vi "R30_1-FPGA.vi"() -> ()   [LabVIEW 2016]
uses:
  Glassman Control.ctl
  Faraday Cup Readback.ctl
  Aperture Readback.ctl
  Gate Valve Readback.ctl
  Glassman Readback.ctl
  <vilib>/LabVIEW Targets/FPGA/cRIO/shared/nicrio_ModuleControls/nicrio_cRIO-9871_BaudRateEnum.ctl
  <vilib>/LabVIEW Targets/FPGA/cRIO/shared/nicrio_ModuleControls/nicrio_cRIO-9871_ParityEnum.ctl
  <vilib>/LabVIEW Targets/FPGA/cRIO/shared/nicrio_ModuleControls/nicrio_cRIO-9871_StopBitsEnum.ctl
  <vilib>/LabVIEW Targets/FPGA/cRIO/shared/nicrio_ModuleControls/nicrio_cRIO-9871_DataBitsEnum.ctl
  <vilib>/Platform/TimedLoop/XDataNode/timing_clust.ctl
  <vilib>/Platform/TimedLoop/XDataNode/nitl_modes.ctl
  <vilib>/Platform/TimedLoop/XDataNode/wakeup.ctl
  <vilib>/rvi/FXPMathLib/basic elements/FxpIntAccumulator/subVIs/nifxpmath_IntAccumulator_SimConfig.ctl
  <vilib>/rvi/Emulation/niFpgaGetClockAttributes.vi
  <vilib>/rvi/Emulation/niFpgaSctlEmulationGetInTimedLoop.vi
  <vilib>/rvi/Emulation/niFpgaEmulationReportErrorSimple.vi
  <vilib>/rvi/eio/common/nirviEmuTemplateMethod_errors.vi
  <vilib>/rvi/Analysis/common/codeGenErrors/XNode/niFpgaXNodeCodeGenErrorHandle.vi
  <vilib>/rvi/Emulation/niFpgaCriticalErrorInLSC.vi
  <vilib>/rvi/FXPMathLib/basic elements/FxpIntAccumulator/simVIs/DllFxpIntAccumulator_sub.vi
  <vilib>/rvi/eio/common/nirviEmuTemplatePropertySet_errors.vi
  <vilib>/eio/EIONode/EIONode.xnode
  <vilib>/rvi/Analysis/measure/dc-rms/XNode/niFpgaDC-RMS.xnode
  <vilib>/Platform/TimedLoop/XDataNode/XDataNode.xnode
  <vilib>/rvi/FXPMathLib/basic elements/FxpIntAccumulator/XNode/nifxpmath_IntAccumulator.xnode
  <vilib>/rvi/FXPMathLib/FxpMul/XNode/nifxpmath_Multiplier.xnode
  <vilib>/eio/EIOPropertyNode/EIOPropertyNode.xnode
  <vilib>/eio/EIOMethodNode/EIOMethodNode.xnode
  <vilib>/Platform/TimedLoop/XDataNode/XDNodeRunTimeDep.lvlib
  <vilib>/rvi/FXPMathLib/sim/FxpSim.dll
  <vilib>/rvi/eio/common/nirviEmuTemplatePropertyGet_errors.vi
  <vilib>/rvi/eio/common/nirviEmuTemplatePropertyGet_noerrors.vi
  <vilib>/rvi/eio/common/nirviEmuTemplatePropertySet_noerrors.vi
panel:
  in  "Switch Obj Vac interlock bypass":bool
  in  "Vac cluster 3 interlock bypass":bool
  in  "Vac cluster 2 interlock bypass":bool
  in  "Vac cluster 1 interlock bypass":bool
  in  "Switch Object Vac Interlock":bool
  out "HV readback loop error":errorcluster
  out "Quad B I read":fxp<+/-,26,5>
  out "Quad A I read":fxp<+/-,26,5>
  out "ESA- Monitor":T1
  out "Mag Steerer Monitor":T1
  out "Y- Steerer Monitor":T1
  out "ESA+ Monitor":T1
  out "X+ Steerer Monitor":T1
  out "X- Steerer Monitor":T1
  out "Y+ Steerer Monitor":T1
  in  "RT error":bool
  out "GV Interlock loop error":errorcluster
  out "Vac cluster 3 Interlock":bool
  out "Vac cluster 2 Interlock":bool
  out "Vac cluster 1 Interlock":bool
  in  "Turbo 2 GV Actuator":bool
  in  "Beamline GV 2 Actuator":bool
  in  "Cryo Pump GV Actuator":bool
  in  "Beamline GV 1 Actuator":bool
  in  "Turbo 1 GV Actuator":bool
  in  "Switch Magnet GV Actuator":bool
  out "GV Status Loop error":errorcluster
  out "Cryo Pump GV Status":T2
  out "Turbo 2 GV Status":T2
  out "Beamline GV 2 Status":T2
  out "Turbo 1 GV Status":T2
  out "Beamline GV 1 Status":T2
  out "Switching Mag GV Status":T2
  in  "ESA- HV Enable":bool
  in  "ESA+ HV Enable":bool
  out "Switch Magnet Aperture Position":T3
  out "Detector Aperture Position":T3
  out "Detector FC Position":T4
  out "Switch Magnet FC Position":T4
  out "Actuator loop error":errorcluster
  in  "Y- Steerer V set":T5
  in  "Y+ Steerer V set":T5
  in  "X- Steerer V set":T5
  in  "X+ Steerer V set":T5
  in  "Quad B set":fxp<+/-,20,5>
  in  "Quad A set":fxp<+/-,20,5>
  in  "ESA Voltage set":fxp<+/-,20,5>
  out "HV control loop error":errorcluster
  out "Cryo Readback error":errorcluster
  out "Vacuum Gauge 1 error":errorcluster
  out "Vacuum Gauge 2 error":errorcluster
  out "Vacuum Gauge 3 error":errorcluster
  out "Switch Image Ion Gauge 1":u8[](array[numeric])
  out "Switch Image Convectron 1":u8[](array[numeric])
  out "Time since repurge":u8[](array[numeric])
  out "1st stage temp":u8[](array[numeric])
  out "2nd stage temp":u8[](array[numeric])
  out "Cryo On-time":u8[](array[numeric])
  out "Cryo Status":u8[](array[numeric])
  out "R30 ESA Convectron  1":u8[](array[numeric])
  out "R30 ESA Ion gauge 1":u8[](array[numeric])
  out "R30 Detector Convectron  1":u8[](array[numeric])
  out "R30 Detector Ion gauge 1":u8[](array[numeric])
  in  "Mag Steerer I-program":fxp<+/-,20,5> format="%.17g"
  in  "Switch magnet Aperture Actuator":bool
  in  "Detector Aperture Actuator":bool
  in  "Detector FC Actuator":bool
  in  "Switch magnet FC Actuator":bool
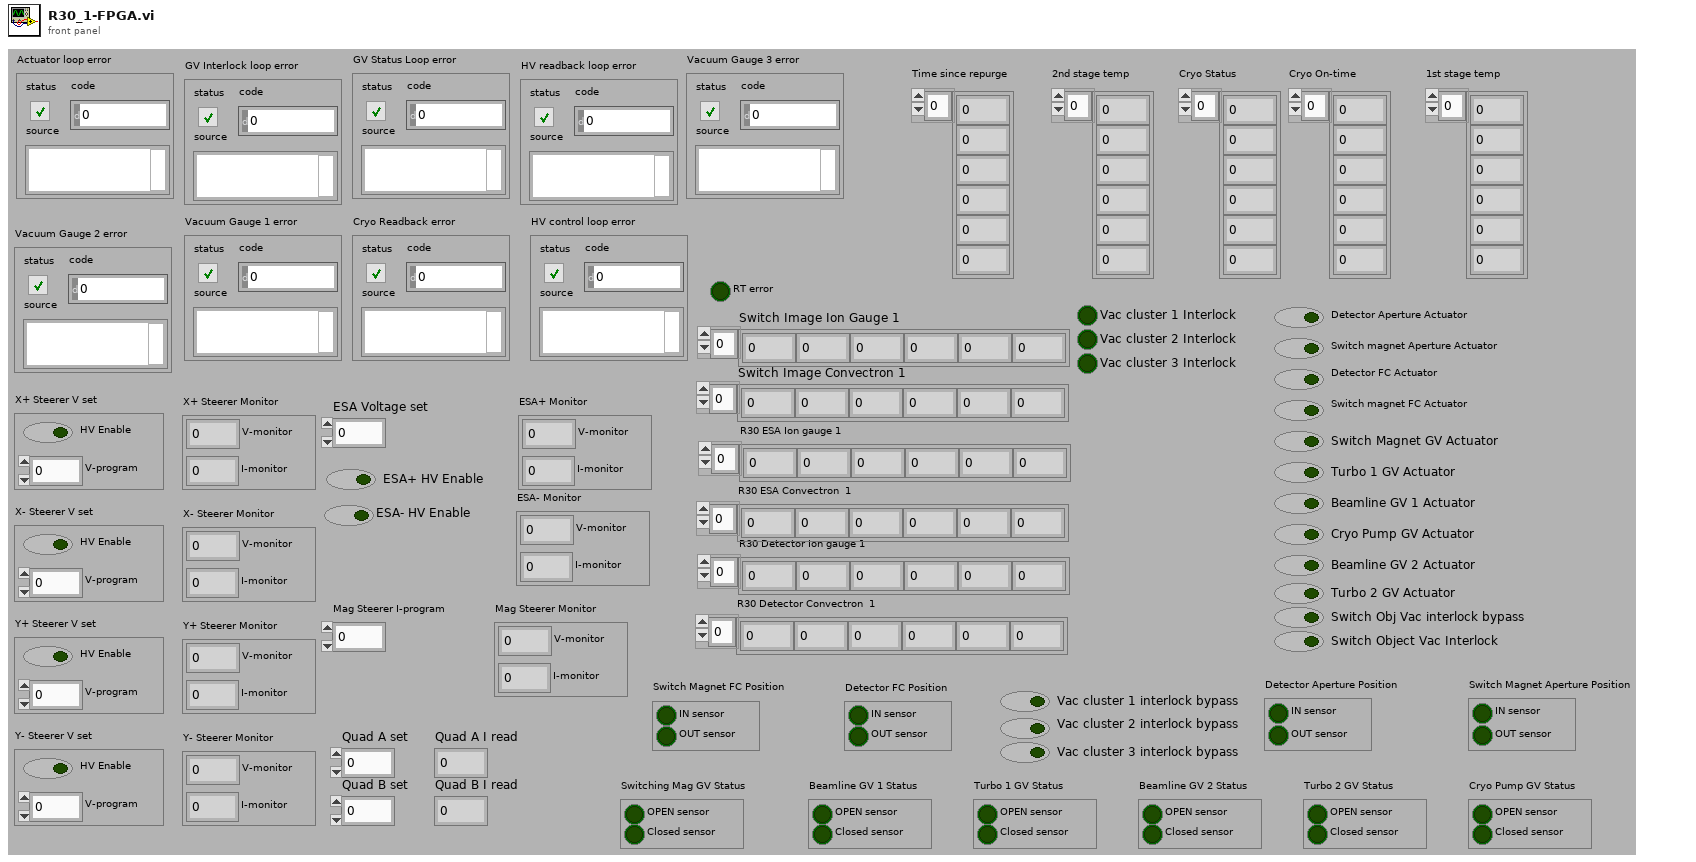
[diagram p1: front panel]
types:
  T1 = typedef "Glassman Readback.ctl" = cluster{"I-monitor":fxp<+/-,16,5>, "V-monitor":fxp<+/-,16,5>}
  T2 = typedef "Gate Valve Readback.ctl" = cluster{"OPEN sensor":bool, "Closed sensor":bool}
  T3 = typedef "Aperture Readback.ctl" = cluster{"IN sensor":bool, "OUT sensor":bool}
  T4 = typedef "Faraday Cup Readback.ctl" = cluster{"IN sensor":bool, "OUT sensor":bool}
  T5 = typedef "Glassman Control.ctl" = cluster{"V-program":fxp<+/-,16,5>, "HV Enable":bool}
  T6 = typedef "nicrio_cRIO-9871_StopBitsEnum.ctl" = enum8{"1", "1.5", "2"}
  T7 = typedef "nicrio_cRIO-9871_ParityEnum.ctl" = enum8{"None", "Odd", "Even", "Mark", "Space"}
  T8 = typedef "nicrio_cRIO-9871_DataBitsEnum.ctl" = enum8{"5", "6", "7", "8"}
  T9 = typedef "nicrio_cRIO-9871_BaudRateEnum.ctl" = enum16{"75 bps", "110 bps", "134 bps", "150 bps", "300 bps", "600 bps", "1200 bps", "1800 bps", "2400 bps", "4800 bps", "7200 bps", "9600 bps", "14.4 kbps", "19.2 kbps", "28.8 kbps", "38.4 kbps", "57.6 kbps", "115.2 kbps", "230.4 kbps", "460.8 kbps", "921.6 kbps"}
  T10 = typedef "XDNodeRunTimeDep.lvlib/timing_clust.ctl" = cluster{"Expected End [f-1]":u64, "Actual End [f-1]":u64, "Finished Late? [f-1]":bool, "Expected End [i-1]":u64, "Actual End [i-1]":u64, "Finished Late? [i-1]":bool, "Expected Start [i]":u64, "Actual Start [i]":u64, "Expected Start [f]":u64, "Actual Start [f]":u64, "Source Name":string, "Structure Name":string, "Period":i64, "Deadline":i64, "Offset":i64, "Start":i64, "Priority":i32, "Timeout":i32, "Mode":T11, "Wakeup Reason":T12, "Error":errorcluster, "Source Type":string, "Secondary Source Type":string, "Global End Time":u64, "Global Start Time":u64, "Frame Duration":u64, "Iteration Duration":u64, "Assigned CPU":i32, "I/O Scan Engine Mode":u32}
  T11 = typedef "XDNodeRunTimeDep.lvlib/nitl_modes.ctl" = enum32{"No Change", "Process missed periods, maintain original phase", "Discard missed periods, maintain original phase", "Process missed periods, ignore original phase", "Discard missed periods, ignore original phase"}
  T12 = typedef "XDNodeRunTimeDep.lvlib/wakeup.ctl" = enum32{"Normal", "Aborted", "Asynchronous wakeup", "Timing source error", "Timed loop error", "Timeout"}
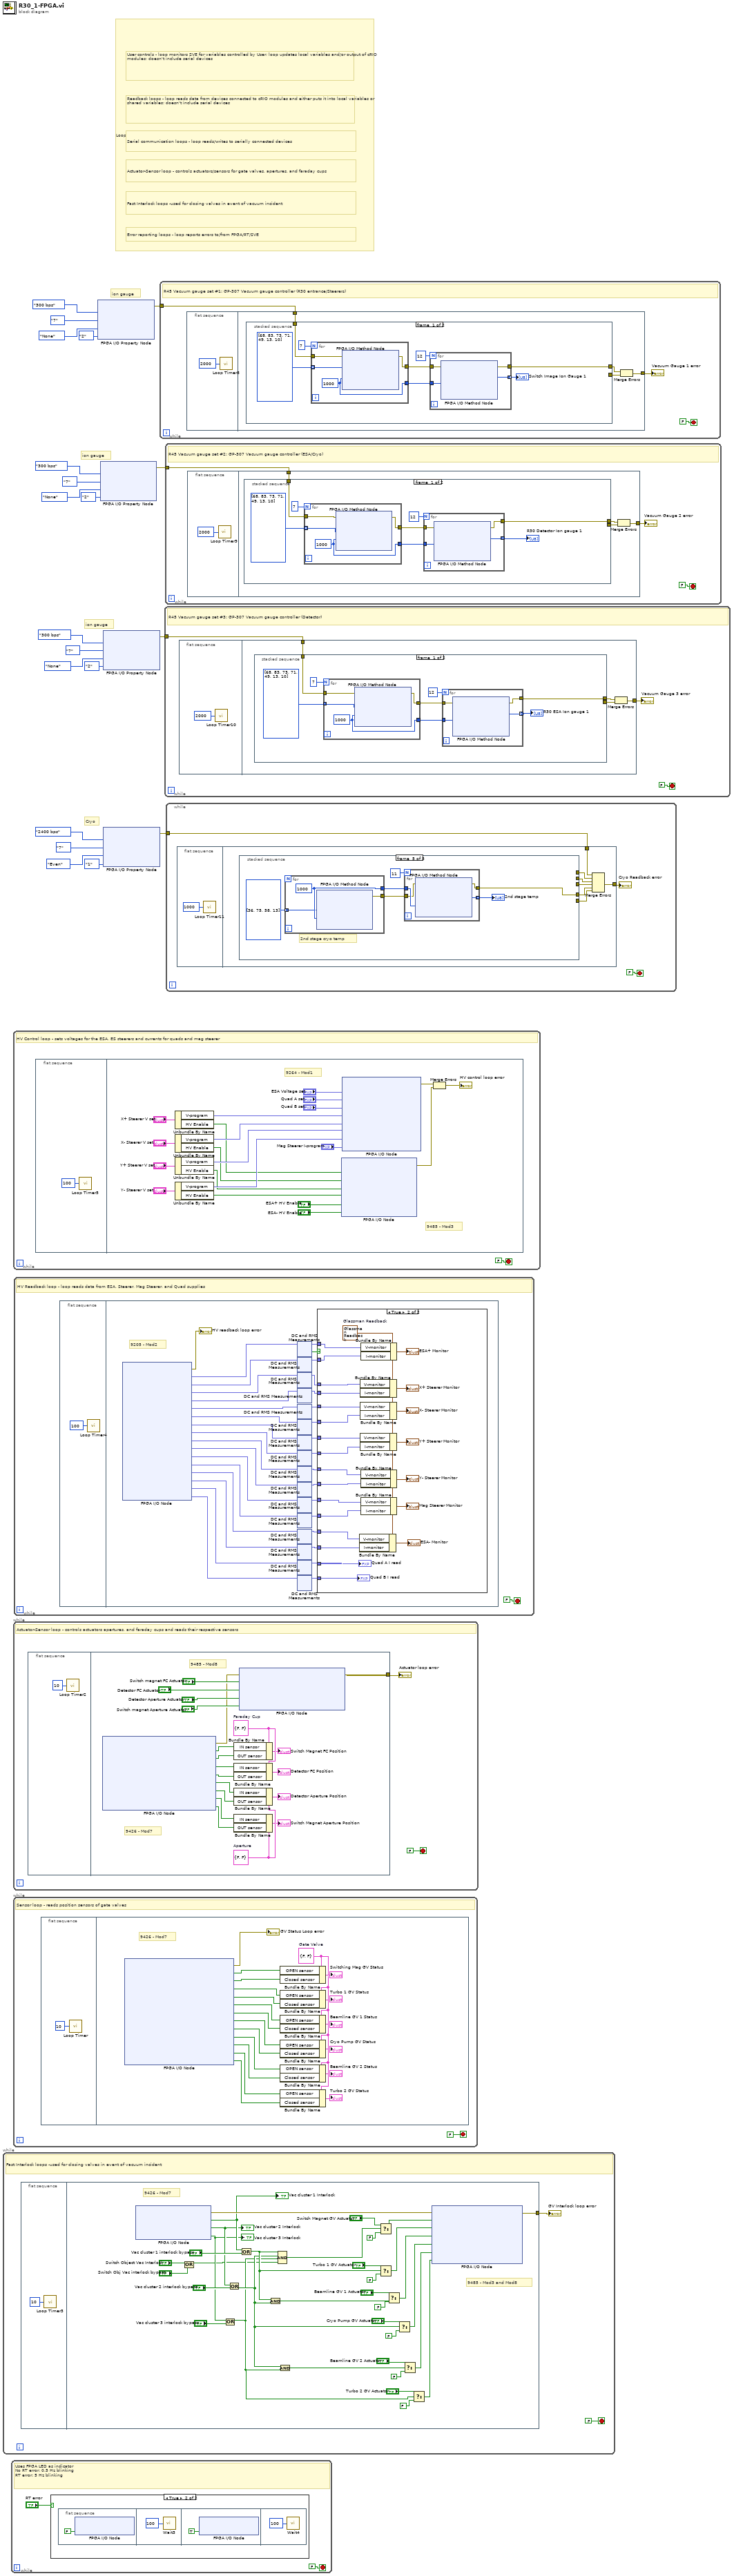
[diagram p0: block diagram]
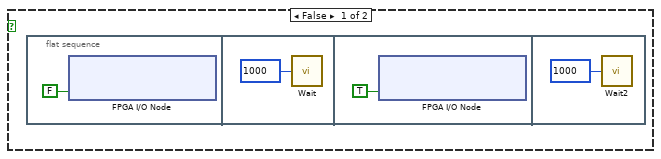
[diagram p2: hidden frame]
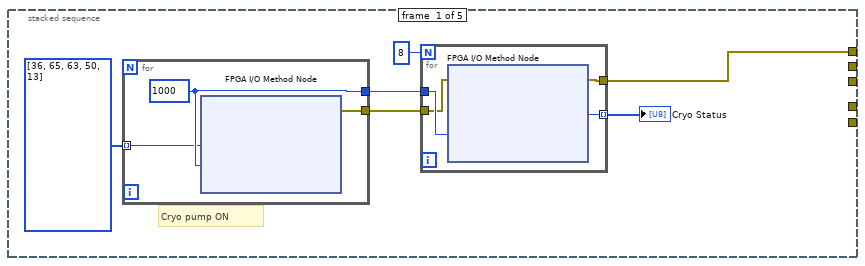
[diagram p3: hidden frame]
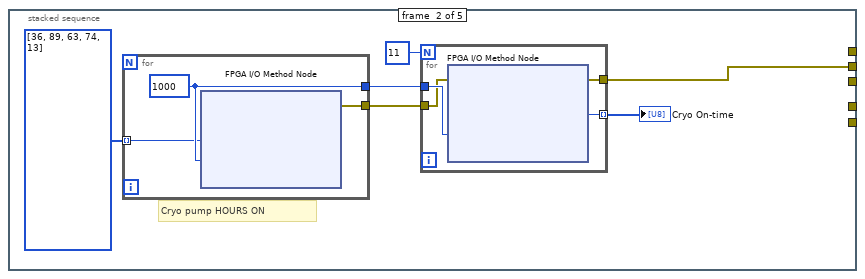
[diagram p4: hidden frame]
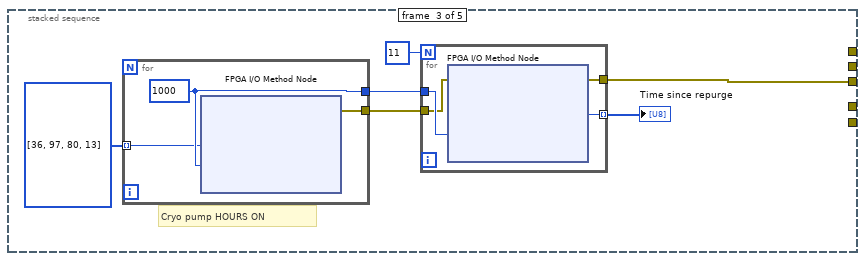
[diagram p5: hidden frame]
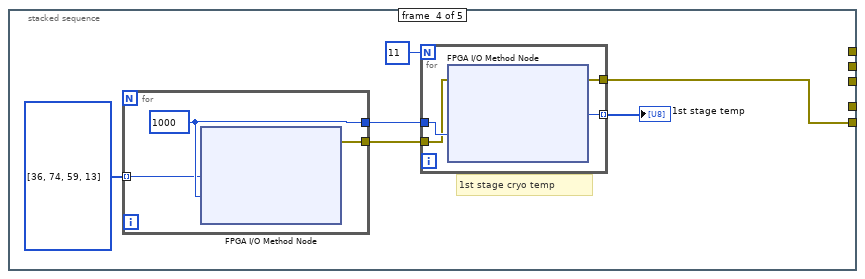
[diagram p6: hidden frame]
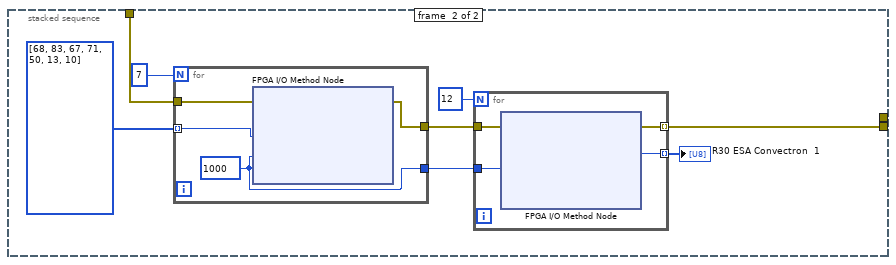
[diagram p7: hidden frame]
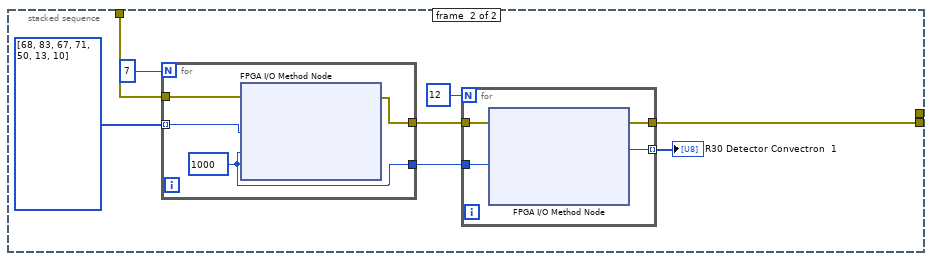
[diagram p8: hidden frame]
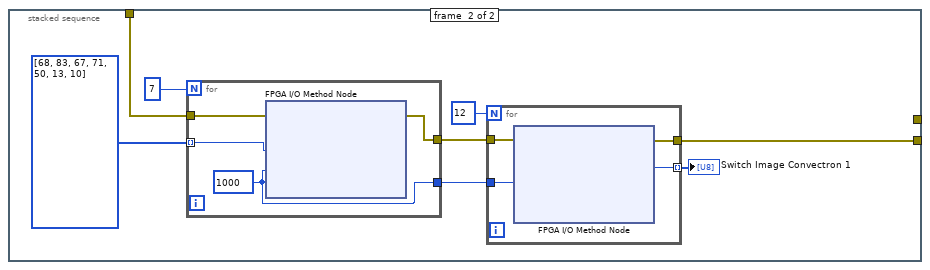
[diagram p9: hidden frame]
diagram:
  # "Actuator-Sensor loop - controls actuators/sensors for gate valves, apertures, and faraday cups"
  # "Fast Interlock loops -used for closing valves in event of vacuum incident"
  # "Error reporting loops - loop reports errors to/from FPGA/RT/SVE"
  # "Serial communication loops - loop reads/writes to serially connected devices"
  # "Readback loops - loop reads data from devices connected to cRIO modules and either puts it into local variables or shared variables; doesn't include serial devices"
  # "User controls - loop monitors SVE for variables controlled by User; loop updates local variables and/or output of cRIO modules; doesn't include serial devices"
  # "Loop legend - loops are color coded by responsibility"
  # "Cryo"
  # "ion gauge"
  # "ion gauge"
  # "ion gauge"
  n1 = while {
    stop <- FALSE stop-if-true
    # "Fast Interlock loops -used for closing valves in event of vacuum incident"
    n2 = flat-sequence {
      tunnel: [w36] -> w21
      frame #0 {
        n3 = call "Loop Timer3"("Count(uSec)"=u32 10) -> ()  [unwired: 1 out]
      }
      frame #1 {
        # "9485 - Mod3 and Mod8"
        # "9426 - Mod7"
        n4 = xnode "FPGA I/O Node"() -> ("error out"=w58:errorcluster, "Vac cluster 1 Interlock"=w33:bool, "Vac cluster 2 Interlock"=w30:bool, "Vac cluster 3 Interlock"=w28:bool)  [unwired: 4 in, 3 out]
        "Vac cluster 1 Interlock" <- w33
        "Vac cluster 2 Interlock" <- w30
        "Vac cluster 3 Interlock" <- w28
        n5 = Or(x="Switch Object Vac Interlock", y="Switch Obj Vac interlock bypass") -> (x .or. y?=w25:bool)
        n6 = Or(x=w28, y="Vac cluster 3 interlock bypass") -> (x .or. y?=w27:bool)
        n7 = Or(x=w30, y="Vac cluster 2 interlock bypass") -> (x .or. y?=w31:bool)
        n8 = Or(x=w33, y="Vac cluster 1 interlock bypass") -> (x .or. y?=w34:bool)
        n9 = And(x=w34, y=w31) -> (x .and. y?=w44:bool)
        n10 = Compound Arithmetic op=AND(w34, w31, w27, w25) -> (w38:bool)
        n11 = And(x=w31, y=w27) -> (x .and. y?=w51:bool)
        n12 = Select(t="Switch Magnet GV Actuator", s=w38, f=FALSE) -> (s? t:f=w37:bool)
        n13 = Select(t="Turbo 1 GV Actuator", s=w34, f=FALSE) -> (s? t:f=w42:bool)
        n14 = Select(t="Beamline GV 1 Actuator", s=w44, f=FALSE) -> (s? t:f=w46:bool)
        n15 = Select(t="Cryo Pump GV Actuator", s=w31, f=FALSE) -> (s? t:f=w49:bool)
        n16 = Select(t="Beamline GV 2 Actuator", s=w51, f=FALSE) -> (s? t:f=w53:bool)
        n17 = Select(t="Turbo 2 GV Actuator", s=w27, f=FALSE) -> (s? t:f=w56:bool)
        n18 = xnode "FPGA I/O Node"("error in"=w58, "Switch Magnet GV Actuator"=w37, "Turbo 1 GV Actuator"=w42, "Beamline GV 1 Actuator"=w46, "Cryo Pump GV Actuator"=w49, "Beamline GV 2 Actuator"=w53, "Turbo 2 GV Actuator"=w56) -> ("error out"=w36:errorcluster)  [unwired: 6 in, 6 out]
      }
    }
    "GV Interlock loop error" <- w21
  }
  n19 = while {
    stop <- FALSE stop-if-true
    # "Uses FPGA LED as indicator\nNo RT error: 0.5 Hz blinking\nRT error: 5 Hz blinking"
    n20 = case shown="True" "RT error" {
      frame False {
        n21 = flat-sequence {
          frame #0 {
            n22 = xnode "FPGA I/O Node"("USER FPGA LED"=FALSE ("FPGA LED")) -> ()  [unwired: 1 in, 1 out]
          }
          frame #1 {
            n23 = call "Wait"("Count(mSec)"=u16 1000) -> ()  [unwired: 1 out]
          }
          frame #2 {
            n24 = xnode "FPGA I/O Node"("USER FPGA LED"=TRUE ("FPGA LED")) -> ()  [unwired: 1 in, 1 out]
          }
          frame #3 {
            n25 = call "Wait2"("Count(mSec)"=u16 1000) -> ()  [unwired: 1 out]
          }
        }
      }
      frame True {
        n26 = flat-sequence {
          frame #0 {
            n27 = xnode "FPGA I/O Node"("USER FPGA LED"=FALSE ("FPGA LED")) -> ()  [unwired: 1 in, 1 out]
          }
          frame #1 {
            n28 = call "Wait3"("Count(mSec)"=u16 100) -> ()  [unwired: 1 out]
          }
          frame #2 {
            n29 = xnode "FPGA I/O Node"("USER FPGA LED"=TRUE ("FPGA LED")) -> ()  [unwired: 1 in, 1 out]
          }
          frame #3 {
            n30 = call "Wait4"("Count(mSec)"=u16 100) -> ()  [unwired: 1 out]
          }
        }
      }
    }
  }
  n31 = while {
    stop <- FALSE stop-if-true
    # "Actuator-Sensor loop - controls actuators apertures, and faraday cups and reads their respective sensors"
    n32 = flat-sequence {
      tunnel: [w89] -> w69
      frame #0 {
        n33 = call "Loop Timer2"("Count(uSec)"=u32 10) -> ()  [unwired: 1 out]
      }
      frame #1 {
        w78 = T3 {"IN sensor"=FALSE, "OUT sensor"=FALSE}  # Aperture
        w81 = T4 {"IN sensor"=FALSE, "OUT sensor"=FALSE}  # Faraday Cup
        # "9485 - Mod8"
        # "9426 - Mod7"
        n34 = xnode "FPGA I/O Node"() -> ("error out"=w86:errorcluster, "Switch Magnet FC IN sensor"=w85:bool, "Switch Magnet FC OUT sensor"=w84:bool, "Detector FC IN sensor"=w83:bool, "Detector FC OUT sensor"=w82:bool, "Detector Aperture IN sensor"=w74:bool, "Detector Aperture OUT sensor"=w75:bool, "Switch Magnet Aperture IN sensor"=w76:bool, "Switch Magnet Aperture OUT sensor"=w77:bool)  [unwired: 9 in, 8 out]
        n35 = Bundle By Name(cluster=w81, "IN sensor"=w85, "OUT sensor"=w84) -> (→"Switch Magnet FC Position":T4)
        n36 = Bundle By Name(cluster=w81, "IN sensor"=w83, "OUT sensor"=w82) -> (→"Detector FC Position":T4)
        n37 = Bundle By Name(cluster=w78, "IN sensor"=w74, "OUT sensor"=w75) -> (→"Detector Aperture Position":T3)
        n38 = Bundle By Name(cluster=w78, "IN sensor"=w76, "OUT sensor"=w77) -> (→"Switch Magnet Aperture Position":T3)
        n39 = xnode "FPGA I/O Node"("error in"=w86, "Switch Magnet FC Actuator"="Switch magnet FC Actuator", "Detector FC Actuator"="Detector FC Actuator", "Detector Aperture Actuator"="Detector Aperture Actuator", "Switch Magnet Aperture Actuator"="Switch magnet Aperture Actuator") -> ("error out"=w89:errorcluster)  [unwired: 4 in, 4 out]
      }
    }
    "Actuator loop error" <- w69
  }
  n40 = while {
    stop <- FALSE stop-if-true
    # "Sensor loop - reads position sensors of gate valves"
    n41 = flat-sequence {
      frame #0 {
        n42 = call "Loop Timer"("Count(uSec)"=u32 10) -> ()  [unwired: 1 out]
      }
      frame #1 {
        w112 = T2 {"OPEN sensor"=FALSE, "Closed sensor"=FALSE}  # Gate Valve
        # "9426 - Mod7"
        n43 = xnode "FPGA I/O Node"() -> ("error out"=→"GV Status Loop error":errorcluster, "Swtich Magnet GV OPEN Sensor"=w111:bool, "Swtich Magnet GV CLOSED Sensor"=w110:bool, "Turbo 1 GV OPEN sensor"=w109:bool, "Turbo 1 GV CLOSED sensor"=w108:bool, "Beamline GV 1 OPEN sensor"=w107:bool, "Beamline GV 1 CLOSED sensor"=w106:bool, "Cryo Pump GV OPEN sensor"=w105:bool, "Cryo Pump GV CLOSED sensor"=w104:bool, "Beamline GV 2 OPEN sensor"=w103:bool, "Beamline GV 2 CLOSED sensor"=w102:bool, "Turbo 2 GV OPEN sensor"=w101:bool, "Turbo 2 GV CLOSED sensor"=w100:bool)  [unwired: 13 in, 12 out]
        n44 = Bundle By Name(cluster=w112, "OPEN sensor"=w111, "Closed sensor"=w110) -> (→"Switching Mag GV Status":T2)
        n45 = Bundle By Name(cluster=w112, "OPEN sensor"=w109, "Closed sensor"=w108) -> (→"Turbo 1 GV Status":T2)
        n46 = Bundle By Name(cluster=w112, "OPEN sensor"=w107, "Closed sensor"=w106) -> (→"Beamline GV 1 Status":T2)
        n47 = Bundle By Name(cluster=w112, "OPEN sensor"=w105, "Closed sensor"=w104) -> (→"Cryo Pump GV Status":T2)
        n48 = Bundle By Name(cluster=w112, "OPEN sensor"=w103, "Closed sensor"=w102) -> (→"Beamline GV 2 Status":T2)
        n49 = Bundle By Name(cluster=w112, "OPEN sensor"=w101, "Closed sensor"=w100) -> (→"Turbo 2 GV Status":T2)
      }
    }
  }
  n50 = while {
    stop <- FALSE stop-if-true
    # "HV Control loop - sets voltages for the ESA, ES steerers and currents for quads and mag steerer"
    n51 = flat-sequence {
      frame #0 {
        n52 = call "Loop Timer5"("Count(mSec)"=u32 100) -> ()  [unwired: 1 out]
      }
      frame #1 {
        # "9264 - Mod1"
        # "9485 - Mod3"
        n53 = Unbundle By Name("X+ Steerer V set") -> ("V-program"=w127:fxp<+/-,16,5>, "HV Enable"=w120:bool)
        n54 = Unbundle By Name("X- Steerer V set") -> ("V-program"=w126:fxp<+/-,16,5>, "HV Enable"=w121:bool)
        n55 = Unbundle By Name("Y+ Steerer V set") -> ("V-program"=w125:fxp<+/-,16,5>, "HV Enable"=w122:bool)
        n56 = Unbundle By Name("Y- Steerer V set") -> ("V-program"=w124:fxp<+/-,16,5>, "HV Enable"=w123:bool)
        n57 = xnode "FPGA I/O Node"("X+ Steerer HV Enable"=w120, "X- Steerer HV Enable"=w121, "Y+ Steerer HV Enable"=w122, "Y- Steerer HV Enable"=w123, "ESA+ HV Enable"="ESA+ HV Enable", "ESA- HV Enable"="ESA- HV Enable") -> ("error out"=w118:errorcluster)  [unwired: 7 in, 6 out]
        n58 = xnode "FPGA I/O Node"("ESA Voltage set"="ESA Voltage set", "Quad A set"="Quad A set", "Quad B set"="Quad B set", "X+ Steerer V set"=w127, "X- Steerer V set"=w126, "Y+ Steerer V set"=w125, "Y- Steerer V set"=w124, "Mag Steerer I-program"="Mag Steerer I-program") -> ("error out"=w135:errorcluster)  [unwired: 9 in, 8 out]
        n59 = Merge Errors(w135, w118) -> (→"HV control loop error":errorcluster)
      }
    }
  }
  n60 = while {
    stop <- FALSE stop-if-true
    # "HV Readback loop - loop reads data from ESA, Steerer, Mag Steerer, and Quad supplies"
    n61 = flat-sequence {
      frame #0 {
        n62 = call "Loop Timer4"("Count(mSec)"=u32 100 ("Count(Ticks)")) -> ()  [unwired: 1 out]
      }
      frame #1 {
        # "9205 - Mod2"
        n63 = xnode "FPGA I/O Node"() -> ("error out"=→"HV readback loop error":errorcluster, "ESA+ V read"=w163:fxp<+/-,26,5>, "ESA+ I read"=w162:fxp<+/-,26,5>, "X+ Steerer V read"=w161:fxp<+/-,26,5>, "X+ Steerer I read"=w160:fxp<+/-,26,5>, "X- Steerer V read"=w159:fxp<+/-,26,5>, "X- Steerer I read"=w158:fxp<+/-,26,5>, "Y+ Steerer V read"=w157:fxp<+/-,26,5>, "Y+ Steerer I read"=w156:fxp<+/-,26,5>, "Y- Steerer V read"=w149:fxp<+/-,26,5>, "Y- Steerer I read"=w148:fxp<+/-,26,5>, "Mag Steerer V read"=w147:fxp<+/-,26,5>, "Mag Steerer I read"=w146:fxp<+/-,26,5>, "ESA- V read"=w145:fxp<+/-,26,5>, "ESA- I read"=w144:fxp<+/-,26,5>, "Quad A I read"=w143:fxp<+/-,26,5>, "Quad B I read"=w142:fxp<+/-,26,5>)  [unwired: 17 in, 16 out]
        n64 = xnode "DC and RMS Measurements"("input data"=w163) -> ("DC"=w171:fxp<+/-,26,5>, "output valid"=w172:bool)  [unwired: 1 in]
        n65 = xnode "DC and RMS Measurements"("input data"=w162) -> ("DC"=w170:fxp<+/-,26,5>)  [unwired: 1 in, 1 out]
        n66 = xnode "DC and RMS Measurements"("input data"=w161) -> ("DC"=w169:fxp<+/-,26,5>)  [unwired: 1 in, 1 out]
        n67 = xnode "DC and RMS Measurements"("input data"=w160) -> ("DC"=w168:fxp<+/-,26,5>)  [unwired: 1 in, 1 out]
        n68 = xnode "DC and RMS Measurements"("input data"=w159) -> ("DC"=w167:fxp<+/-,26,5>)  [unwired: 1 in, 1 out]
        n69 = xnode "DC and RMS Measurements"("input data"=w158) -> ("DC"=w166:fxp<+/-,26,5>)  [unwired: 1 in, 1 out]
        n70 = xnode "DC and RMS Measurements"("input data"=w157) -> ("DC"=w165:fxp<+/-,26,5>)  [unwired: 1 in, 1 out]
        n71 = xnode "DC and RMS Measurements"("input data"=w156) -> ("DC"=w164:fxp<+/-,26,5>)  [unwired: 1 in, 1 out]
        n72 = xnode "DC and RMS Measurements"("input data"=w149) -> ("DC"=w155:fxp<+/-,26,5>)  [unwired: 1 in, 1 out]
        n73 = xnode "DC and RMS Measurements"("input data"=w148) -> ("DC"=w154:fxp<+/-,26,5>)  [unwired: 1 in, 1 out]
        n74 = xnode "DC and RMS Measurements"("input data"=w147) -> ("DC"=w153:fxp<+/-,26,5>)  [unwired: 1 in, 1 out]
        n75 = xnode "DC and RMS Measurements"("input data"=w146) -> ("DC"=w152:fxp<+/-,26,5>)  [unwired: 1 in, 1 out]
        n76 = xnode "DC and RMS Measurements"("input data"=w145) -> ("DC"=w151:fxp<+/-,26,5>)  [unwired: 1 in, 1 out]
        n77 = xnode "DC and RMS Measurements"("input data"=w144) -> ("DC"=w150:fxp<+/-,26,5>)  [unwired: 1 in, 1 out]
        n78 = xnode "DC and RMS Measurements"("input data"=w143) -> ("DC"=w141:fxp<+/-,26,5>)  [unwired: 1 in, 1 out]
        n79 = xnode "DC and RMS Measurements"("input data"=w142) -> ("DC"=w140:fxp<+/-,26,5>)  [unwired: 1 in, 1 out]
        n80 = case shown="True" w172 {
          tunnel: w171 -> [_ w996]
          tunnel: w170 -> [_ w995]
          tunnel: w169 -> [_ w991]
          tunnel: w168 -> [_ w990]
          tunnel: w167 -> [_ w989]
          tunnel: w166 -> [_ w988]
          tunnel: w165 -> [_ w986]
          tunnel: w164 -> [_ w985]
          tunnel: w155 -> [_ w981]
          tunnel: w154 -> [_ w980]
          tunnel: w153 -> [_ w979]
          tunnel: w152 -> [_ w978]
          tunnel: w151 -> [_ w977]
          tunnel: w150 -> [_ w976]
          tunnel: w141 -> [_ w974]
          tunnel: w140 -> [_ w973]
          frame False {
          }
          frame True {
            w975 = T1 {"I-monitor"=0.0, "V-monitor"=0.0}  # Glassman Readback
            n81 = Bundle By Name(cluster=w975, "V-monitor"=w977, "I-monitor"=w976) -> (→"ESA- Monitor":T1)
            n82 = Bundle By Name(cluster=w975, "V-monitor"=w991, "I-monitor"=w990) -> (→"X+ Steerer Monitor":T1)
            n83 = Bundle By Name(cluster=w975, "V-monitor"=w989, "I-monitor"=w988) -> (→"X- Steerer Monitor":T1)
            n84 = Bundle By Name(cluster=w975, "V-monitor"=w986, "I-monitor"=w985) -> (→"Y+ Steerer Monitor":T1)
            n85 = Bundle By Name(cluster=w975, "V-monitor"=w996, "I-monitor"=w995) -> (→"ESA+ Monitor":T1)
            n86 = Bundle By Name(cluster=w975, "V-monitor"=w981, "I-monitor"=w980) -> (→"Y- Steerer Monitor":T1)
            n87 = Bundle By Name(cluster=w975, "V-monitor"=w979, "I-monitor"=w978) -> (→"Mag Steerer Monitor":T1)
            "Quad A I read" <- w974
            "Quad B I read" <- w973
          }
        }
      }
    }
  }
  n88 = xnode "FPGA I/O Property Node"("Baud Rate"=nicrio_cRIO-9871_BaudRateEnum."300 bps", "Data Bits"=nicrio_cRIO-9871_DataBitsEnum."7", "Parity"=nicrio_cRIO-9871_ParityEnum."None", "Stop Bits"=nicrio_cRIO-9871_StopBitsEnum."2") -> ("error out"=w4:errorcluster)  [unwired: 2 in, 1 out]
  n89 = xnode "FPGA I/O Property Node"("Baud Rate"=nicrio_cRIO-9871_BaudRateEnum."300 bps", "Data Bits"=nicrio_cRIO-9871_DataBitsEnum."7", "Parity"=nicrio_cRIO-9871_ParityEnum."None", "Stop Bits"=nicrio_cRIO-9871_StopBitsEnum."2") -> ("error out"=w3:errorcluster)  [unwired: 2 in, 1 out]
  n90 = xnode "FPGA I/O Property Node"("Baud Rate"=nicrio_cRIO-9871_BaudRateEnum."300 bps", "Data Bits"=nicrio_cRIO-9871_DataBitsEnum."7", "Parity"=nicrio_cRIO-9871_ParityEnum."None", "Stop Bits"=nicrio_cRIO-9871_StopBitsEnum."2") -> ("error out"=w2:errorcluster)  [unwired: 2 in, 1 out]
  n91 = xnode "FPGA I/O Property Node"("Baud Rate"=nicrio_cRIO-9871_BaudRateEnum."2400 bps", "Data Bits"=nicrio_cRIO-9871_DataBitsEnum."7", "Parity"=nicrio_cRIO-9871_ParityEnum."Even", "Stop Bits"=nicrio_cRIO-9871_StopBitsEnum."1") -> ("error out"=w1:errorcluster)  [unwired: 2 in, 1 out]
  n92 = while {
    tunnel: w4 -> [w1478]
    stop <- FALSE stop-if-true
    # "R45 Vacuum gauge set #1: GP-307 Vacuum gauge controller (R30 entrance/Steerers)"
    n93 = flat-sequence {
      tunnel: w1478 -> [w1484]
      tunnel: [w1481] -> w1477
      frame #0 {
        n94 = call "Loop Timer8"("Count(mSec)"=u32 2000 ("Count(Ticks)")) -> ()  [unwired: 1 out]
      }
      frame #1 {
        n95 = stacked-sequence {
          tunnel: w1484 -> [w1487 w1503]
          tunnel: [_ w1501] -> w1483
          tunnel: [w1485 _] -> w1482
          frame #0 {
            n96 = for {
              N: 7 -> [_]
              tunnel: [w1499] -> w1492
              tunnel: u8[] [68, 83, 73, 71, 49, 13, 10] ("unsigned byte array") -> [w1500] mode=indexing
              tunnel: w1487 -> [w1498]
              tunnel: [w1497] -> w1486
              w1499 = 1000 ("Timeout (ms)")
              n97 = xnode "FPGA I/O Method Node"("error in"=w1498, "Data"=w1500, "Timeout (ms)"=w1499) -> ("error out"=w1497:errorcluster)  [unwired: 1 in, 2 out]
            }
            n98 = for {
              N: 12 -> [_]
              tunnel: w1492 -> [w1496]
              tunnel: [w1495] -> w1488 mode=indexing
              tunnel: w1486 -> [w1494]
              tunnel: [w1493] -> w1485
              n99 = xnode "FPGA I/O Method Node"("error in"=w1494, "Timeout (ms)"=w1496) -> ("error out"=w1493:errorcluster, "Data"=w1495:u8)  [unwired: 1 in, 2 out]
            }
            "Switch Image Ion Gauge 1" <- w1488
          }
          frame #1 {
            n100 = for {
              N: 7 -> [_]
              tunnel: [w1515] -> w1508
              tunnel: u8[] [68, 83, 67, 71, 50, 13, 10] ("unsigned byte array") -> [w1516] mode=indexing
              tunnel: w1503 -> [w1514]
              tunnel: [w1513] -> w1502
              w1515 = 1000 ("Timeout (ms)")
              n101 = xnode "FPGA I/O Method Node"("error in"=w1514, "Data"=w1516, "Timeout (ms)"=w1515) -> ("error out"=w1513:errorcluster)  [unwired: 1 in, 2 out]
            }
            n102 = for {
              N: 12 -> [_]
              tunnel: w1508 -> [w1512]
              tunnel: [w1511] -> w1504 mode=indexing
              tunnel: w1502 -> [w1510]
              tunnel: [w1509] -> w1501
              n103 = xnode "FPGA I/O Method Node"("error in"=w1510, "Timeout (ms)"=w1512) -> ("error out"=w1509:errorcluster, "Data"=w1511:u8)  [unwired: 1 in, 2 out]
            }
            "Switch Image Convectron 1" <- w1504
          }
        }
        n104 = Merge Errors(w1482, w1483) -> (w1481:errorcluster)
      }
    }
    "Vacuum Gauge 1 error" <- w1477
  }
  n105 = while {
    tunnel: w2 -> [w1518]
    stop <- FALSE stop-if-true
    # "R45 Vacuum gauge set #3: GP-307 Vacuum gauge controller (Detector)"
    n106 = flat-sequence {
      tunnel: w1518 -> [w1524]
      tunnel: [w1521] -> w1517
      frame #0 {
        n107 = call "Loop Timer10"("Count(mSec)"=u32 2000 ("Count(Ticks)")) -> ()  [unwired: 1 out]
      }
      frame #1 {
        n108 = stacked-sequence {
          tunnel: w1524 -> [w1527 w1543]
          tunnel: [_ w1541] -> w1523
          tunnel: [w1525 _] -> w1522
          frame #0 {
            n109 = for {
              N: 7 -> [_]
              tunnel: [w1539] -> w1532
              tunnel: u8[] [68, 83, 73, 71, 49, 13, 10] ("unsigned byte array") -> [w1540] mode=indexing
              tunnel: w1527 -> [w1538]
              tunnel: [w1537] -> w1526
              w1539 = 1000 ("Timeout (ms)")
              n110 = xnode "FPGA I/O Method Node"("error in"=w1538, "Data"=w1540, "Timeout (ms)"=w1539) -> ("error out"=w1537:errorcluster)  [unwired: 1 in, 2 out]
            }
            n111 = for {
              N: 12 -> [_]
              tunnel: w1532 -> [w1536]
              tunnel: [w1535] -> w1528 mode=indexing
              tunnel: w1526 -> [w1534]
              tunnel: [w1533] -> w1525
              n112 = xnode "FPGA I/O Method Node"("error in"=w1534, "Timeout (ms)"=w1536) -> ("error out"=w1533:errorcluster, "Data"=w1535:u8)  [unwired: 1 in, 2 out]
            }
            "R30 ESA Ion gauge 1" <- w1528
          }
          frame #1 {
            n113 = for {
              N: 7 -> [_]
              tunnel: [w1555] -> w1548
              tunnel: u8[] [68, 83, 67, 71, 50, 13, 10] ("unsigned byte array") -> [w1556] mode=indexing
              tunnel: w1543 -> [w1554]
              tunnel: [w1553] -> w1542
              w1555 = 1000 ("Timeout (ms)")
              n114 = xnode "FPGA I/O Method Node"("error in"=w1554, "Data"=w1556, "Timeout (ms)"=w1555) -> ("error out"=w1553:errorcluster)  [unwired: 1 in, 2 out]
            }
            n115 = for {
              N: 12 -> [_]
              tunnel: w1548 -> [w1552]
              tunnel: [w1551] -> w1544 mode=indexing
              tunnel: w1542 -> [w1550]
              tunnel: [w1549] -> w1541 mode=indexing
              n116 = xnode "FPGA I/O Method Node"("error in"=w1550, "Timeout (ms)"=w1552) -> ("error out"=w1549:errorcluster, "Data"=w1551:u8)  [unwired: 1 in, 2 out]
            }
            "R30 ESA Convectron  1" <- w1544
          }
        }
        n117 = Merge Errors(w1522, w1523) -> (w1521:errorcluster)
      }
    }
    "Vacuum Gauge 3 error" <- w1517
  }
  n118 = while {
    tunnel: w3 -> [w1558]
    stop <- FALSE stop-if-true
    # "R45 Vacuum gauge set #2: GP-307 Vacuum gauge controller (ESA/Cryo)"
    n119 = flat-sequence {
      tunnel: w1558 -> [w1564]
      tunnel: [w1561] -> w1557
      frame #0 {
        n120 = call "Loop Timer9"("Count(mSec)"=u32 2000 ("Count(Ticks)")) -> ()  [unwired: 1 out]
      }
      frame #1 {
        n121 = stacked-sequence {
          tunnel: w1564 -> [w1567 w1583]
          tunnel: [_ w1581] -> w1563
          tunnel: [w1565 _] -> w1562
          frame #0 {
            n122 = for {
              N: 7 -> [_]
              tunnel: [w1579] -> w1572
              tunnel: u8[] [68, 83, 73, 71, 49, 13, 10] ("unsigned byte array") -> [w1580] mode=indexing
              tunnel: w1567 -> [w1578]
              tunnel: [w1577] -> w1566
              w1579 = 1000 ("Timeout (ms)")
              n123 = xnode "FPGA I/O Method Node"("error in"=w1578, "Data"=w1580, "Timeout (ms)"=w1579) -> ("error out"=w1577:errorcluster)  [unwired: 1 in, 2 out]
            }
            n124 = for {
              N: 12 -> [_]
              tunnel: w1572 -> [w1576]
              tunnel: [w1575] -> w1568 mode=indexing
              tunnel: w1566 -> [w1574]
              tunnel: [w1573] -> w1565
              n125 = xnode "FPGA I/O Method Node"("error in"=w1574, "Timeout (ms)"=w1576) -> ("error out"=w1573:errorcluster, "Data"=w1575:u8)  [unwired: 1 in, 2 out]
            }
            "R30 Detector Ion gauge 1" <- w1568
          }
          frame #1 {
            n126 = for {
              N: 7 -> [_]
              tunnel: [w1595] -> w1588
              tunnel: u8[] [68, 83, 67, 71, 50, 13, 10] ("unsigned byte array") -> [w1596] mode=indexing
              tunnel: w1583 -> [w1594]
              tunnel: [w1593] -> w1582
              w1595 = 1000 ("Timeout (ms)")
              n127 = xnode "FPGA I/O Method Node"("error in"=w1594, "Data"=w1596, "Timeout (ms)"=w1595) -> ("error out"=w1593:errorcluster)  [unwired: 1 in, 2 out]
            }
            n128 = for {
              N: 12 -> [_]
              tunnel: w1588 -> [w1592]
              tunnel: [w1591] -> w1584 mode=indexing
              tunnel: w1582 -> [w1590]
              tunnel: [w1589] -> w1581
              n129 = xnode "FPGA I/O Method Node"("error in"=w1590, "Timeout (ms)"=w1592) -> ("error out"=w1589:errorcluster, "Data"=w1591:u8)  [unwired: 1 in, 2 out]
            }
            "R30 Detector Convectron  1" <- w1584
          }
        }
        n130 = Merge Errors(w1562, w1563) -> (w1561:errorcluster)
      }
    }
    "Vacuum Gauge 2 error" <- w1557
  }
  n131 = while {
    tunnel: w1 -> [w1597]
    stop <- FALSE stop-if-true
    n132 = flat-sequence {
      tunnel: [w1602] -> w1598
      tunnel: w1597 -> [w1601]
      frame #0 {
        n133 = call "Loop Timer11"("Count(mSec)"=u32 1000 ("Count(Ticks)")) -> ()  [unwired: 1 out]
      }
      frame #1 {
        n134 = stacked-sequence {
          tunnel: [w1609 _ _ _ _] -> w1607
          tunnel: [_ w1622 _ _ _] -> w1606
          tunnel: [_ _ w1634 _ _] -> w1605
          tunnel: [_ _ _ _ w1660] -> w1604
          tunnel: [_ _ _ w1647 _] -> w1603
          frame #0 {
            # "Cryo pump ON"
            n135 = for {
              tunnel: [w1620] -> w1613
              tunnel: u8[] [36, 65, 63, 50, 13] ("unsigned byte array") -> [w1619] mode=indexing
              tunnel: [w1618] -> w1608
              w1620 = 1000 ("Timeout (ms)")
              n136 = xnode "FPGA I/O Method Node"("Data"=w1619, "Timeout (ms)"=w1620) -> ("error out"=w1618:errorcluster)  [unwired: 2 in, 2 out]
            }
            n137 = for {
              N: 8 -> [_]
              tunnel: w1613 -> [w1617]
              tunnel: [w1616] -> w1610 mode=indexing
              tunnel: [w1615] -> w1609
              tunnel: w1608 -> [w1614]
              n138 = xnode "FPGA I/O Method Node"("error in"=w1614, "Timeout (ms)"=w1617) -> ("error out"=w1615:errorcluster, "Data"=w1616:u8)  [unwired: 1 in, 2 out]
            }
            "Cryo Status" <- w1610
          }
          frame #1 {
            # "Cryo pump HOURS ON"
            n139 = for {
              tunnel: [w1633] -> w1626
              tunnel: u8[] [36, 89, 63, 74, 13] ("unsigned byte array") -> [w1632] mode=indexing
              tunnel: [w1631] -> w1621
              w1633 = 1000 ("Timeout (ms)")
              n140 = xnode "FPGA I/O Method Node"("Data"=w1632, "Timeout (ms)"=w1633) -> ("error out"=w1631:errorcluster)  [unwired: 2 in, 2 out]
            }
            n141 = for {
              N: 11 -> [_]
              tunnel: w1626 -> [w1630]
              tunnel: [w1629] -> w1623 mode=indexing
              tunnel: [w1628] -> w1622
              tunnel: w1621 -> [w1627]
              n142 = xnode "FPGA I/O Method Node"("error in"=w1627, "Timeout (ms)"=w1630) -> ("error out"=w1628:errorcluster, "Data"=w1629:u8)  [unwired: 1 in, 2 out]
            }
            "Cryo On-time" <- w1623
          }
          frame #2 {
            # "Cryo pump HOURS ON"
            n143 = for {
              tunnel: [w1646] -> w1639
              tunnel: u8[] [36, 97, 80, 13] ("unsigned byte array") -> [w1645] mode=indexing
              tunnel: [w1644] -> w1635
              w1646 = 1000 ("Timeout (ms)")
              n144 = xnode "FPGA I/O Method Node"("Data"=w1645, "Timeout (ms)"=w1646) -> ("error out"=w1644:errorcluster)  [unwired: 2 in, 2 out]
            }
            n145 = for {
              N: 11 -> [_]
              tunnel: w1639 -> [w1643]
              tunnel: [w1642] -> w1636 mode=indexing
              tunnel: w1635 -> [w1641]
              tunnel: [w1640] -> w1634
              n146 = xnode "FPGA I/O Method Node"("error in"=w1641, "Timeout (ms)"=w1643) -> ("error out"=w1640:errorcluster, "Data"=w1642:u8)  [unwired: 1 in, 2 out]
            }
            "Time since repurge" <- w1636
          }
          frame #3 {
            # "1st stage cryo temp"
            n147 = for {
              tunnel: [w1659] -> w1652
              tunnel: u8[] [36, 74, 59, 13] ("unsigned byte array") -> [w1658] mode=indexing
              tunnel: [w1657] -> w1648
              w1659 = 1000 ("Timeout (ms)")
              n148 = xnode "FPGA I/O Method Node"("Data"=w1658, "Timeout (ms)"=w1659) -> ("error out"=w1657:errorcluster)  [unwired: 2 in, 2 out]
            }
            n149 = for {
              N: 11 -> [_]
              tunnel: w1652 -> [w1656]
              tunnel: [w1655] -> w1649 mode=indexing
              tunnel: w1648 -> [w1654]
              tunnel: [w1653] -> w1647
              n150 = xnode "FPGA I/O Method Node"("error in"=w1654, "Timeout (ms)"=w1656) -> ("error out"=w1653:errorcluster, "Data"=w1655:u8)  [unwired: 1 in, 2 out]
            }
            "1st stage temp" <- w1649
          }
          frame #4 {
            # "2nd stage cryo temp"
            n151 = for {
              tunnel: [w1672] -> w1665
              tunnel: u8[] [36, 75, 58, 13] ("unsigned byte array") -> [w1671] mode=indexing
              tunnel: [w1670] -> w1661
              w1672 = 1000 ("Timeout (ms)")
              n152 = xnode "FPGA I/O Method Node"("Data"=w1671, "Timeout (ms)"=w1672) -> ("error out"=w1670:errorcluster)  [unwired: 2 in, 2 out]
            }
            n153 = for {
              N: 11 -> [_]
              tunnel: w1665 -> [w1669]
              tunnel: [w1668] -> w1662 mode=indexing
              tunnel: w1661 -> [w1667]
              tunnel: [w1666] -> w1660
              n154 = xnode "FPGA I/O Method Node"("error in"=w1667, "Timeout (ms)"=w1669) -> ("error out"=w1666:errorcluster, "Data"=w1668:u8)  [unwired: 1 in, 2 out]
            }
            "2nd stage temp" <- w1662
          }
        }
        n155 = Merge Errors(w1601, w1607, w1606, w1605, w1604, w1603) -> (w1602:errorcluster)
      }
    }
    "Cryo Readback error" <- w1598
  }
